vi "Check for lock-in 2.vi"() -> (3 "ready?":bool)   [LabVIEW 2009, in "SR830.lvlib"]
doc: "Checks to see if the SR830 lock-in amplifier is available or not by requesting its device ID string."
uses:
  sr830/SR830.lvlib
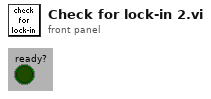
[diagram p1: front panel]
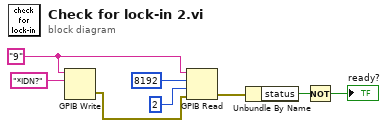
[diagram p0: block diagram]
diagram:
  w7 = "9" ("address string")
  n1 = GPIB Write(0:w7, 1:"*IDN?" ("data")) -> (6:w4:errorcluster)  [unwired: 1 in, 3 out]
  n2 = GPIB Read(0:w7, 1:8192 ("byte count"), 2:i16 2 ("mode (0)"), 3:w4) -> (7:w3:errorcluster)  [unwired: 3 out]
  n3 = Unbundle By Name(w3) -> ("status"=w2:bool)
  n4 = Not(x=w2) -> (.not. x?=→"ready?":bool)
